vi "Default Instrument Setup.vi"(8 "error in (no error)":errorcluster, 11 "VISA resource name":refnum<visa-resource-name>) -> (0 "error out":errorcluster, 3 "VISA resource name out":refnum<visa-resource-name>)   [LabVIEW 2018, in "Agilent PSG MXG Series.lvlib"]
doc: "This Utility VI sends a default command string to the instrument whenever a new VISA session is opened, or the instrument is reset. Use this VI as a subVI for the <B>Initialize</B> and <B>Reset</B> VIs. Altering this VI could cause these two VIs to operate incorrectly."
uses:
  Agilent PSG MXG Series.lvlib
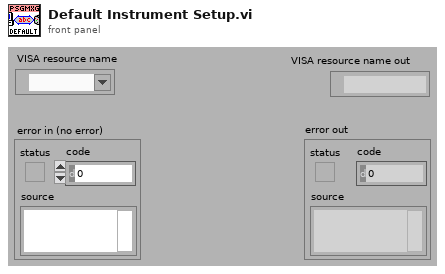
[diagram p1: front panel]
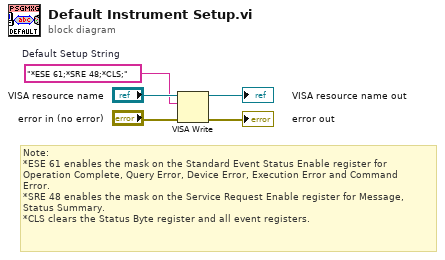
[diagram p0: block diagram]
diagram:
  w1 = "*ESE 61;*SRE 48;*CLS;"  # Default Setup String
  # "Note:\n*ESE 61 enables the mask on the Standard Event Status Enable register for\nOperation Complete, Query Error, Device Error, Execution Error and Command\nError.\n*SRE 48 enables the mask on the Service Request Enable register for Message,\nStatus Summary.\n*CLS clears the Status Byte register and all event registers."
  n1 = VISA Write(VISA resource name="VISA resource name", write buffer=w1, error in (no error)="error in (no error)") -> (VISA resource name out=→"VISA resource name out":refnum<visa-resource-name>, error out=→"error out":errorcluster)  [unwired: 1 out]
